vi "Global_params_reg.vi"() -> ()   [LabVIEW 2019]
uses:
  _ctrl/config_aging.ctl
  Setting_reg.ctl
  Breakdown-Spec.ctl
  _ctrl/DL950_config.ctl
  _ctrl/BP4610_config.ctl
  _ctrl/DSP_config.ctl
  Devices/NI Board/cDAQ-9221 AI/Set_NIAI.ctl
  _ctrl/cDAQ-9269 Config.ctl
  Devices/NI Board/cDAQ-9269 AO/Set_AO_Wave-config.ctl
panel:
  in  "Params_reg-all":T10={"Params"={"Setting"={"제어 전압[V]"=0.0, "출력전압[V]"=0.0, "전류[A]"=0.0, "출력전류[A]"=0.0, "ON[초]"=0.0, "OFF[초]"=0.0, "Irms 허용치 from "=0.0, "Irms 허용치 to"=0.0, "AO Delay ms"=0, "Log"=path "", "result"=path ""}, "TestName"="", "Result path"=path "", "파일 생성 주기[N]"=0, "Test Specs"={"제어단 단선 Irms[mA](이하)"=0.0, "제어단 특성 전류 Irms[mA] Max"=0.0, "제어단 특성 전류 Irms[mA] Min"=0.0, "출력단 단선 Irms[mA](이하)"=0.0, "출력단 특성 전류 Irms[mA]  Max"=0.0, "출력단 특성전류 Irms[mA]  Min"=0.0, "온도[degree]"=0.0}}, "DL950_config"={"Timeout"=10000, "Time Div"=19, "Acq Mode"=0, "Record Len"=5, "Record Num"=0, "Start Point"=0, "End Poin"=60000, "Visa"="TCPIP0::192.168.0.100::inst0::INSTR", "Config Voltage"=[{"Enable"=TRUE, "Ch"=0, "V Div"=12, "Coupling"=1, "Probe"=3, "Act.Items"=FALSE, "items"=[]}, {"Enable"=TRUE, "Ch"=0, "V Div"=12, "Coupling"=1, "Probe"=3, "Act.Items"=FALSE, "items"=[]}], "Trigger on"=FALSE, "Trigger Level"=0.0, "Reset"=FALSE, "Config Temp"=[], "Trig Mode"=1, "Trig Pos"=50.0, "Trigger Slope"=0, "Trigger Source "=1, "Trig Start -5"=-5.0, "End 5"=5.0}, "BP4610 Config"={"VISA"="", "Limit-BP"={"Set"=enum."Current", "Voltage+[V]"=20.0, "Current+[A]"=5.0, "Voltage-[V]"=-20.0, "Current-[A]"=-5.0}, "SET BP"={"Set"=enum."FREQ/WAVE", "Operation mode"=0, "Voltage[Vp-p]"=0.0, "Current[Ap-p]"=0.0, "Voltage[V]"=0.0, "Current[A]"=0.0, "Frequency[Hz]"=1.0, "Waveform"=enum."Sine"}}, "DSP1950 Config"={"Port"="TCPIP0::192.168.0.14::HISLIP0::INSTR", "OVP Level"=0.0, "OCP Level"=0.0, "Current"=0.0, "Voltage"=0.0}, "DMM 2470 Config"={"Source Mode"=enum."Voltage", "Source Limit Level"=0.01, "Source Level"=0.0, "Output_2470"=FALSE}, "cDAQ-9221 Config"={"input terminal"=10083, "minimum value"=-60.0, "maximum value"=60.0, "number of samples"=1000, "rate"=10000.0, "sample mode"=10123, "physical channels"=""}, "cDAQ-9467 Config"="", "cDAQ-9269 AO Config"={"Ch"="cDAQ1Mod1/ao0", "Max V"=5.0, "Min V"=-5.0, " Rate"=1000.0, "N pts"=100, "sample mode"=10178}, "AO_Wave-config"={"offset"=0.0, "Samples"=0, "duty"=0.0, "Rate"=0.0, "wfm"={"Freq"=0.0, "Amp"=0.0, "Type"=enum."Sine Wave"}}} {"cDAQ-9269 AO Config"."sample mode" items=["유한 샘플"=10178, "연속 샘플"=10123, "하드웨어 타이밍에 의한 단일 포인트"=12522]; "cDAQ-9221 Config"."sample mode" items=["Finite Samples"=10178, "Continuous Samples"=10123, "Hardware Timed Single Point"=12522]; "cDAQ-9221 Config"."rate" format="%0.2f"; "cDAQ-9221 Config"."maximum value" format="%^.2e"; "cDAQ-9221 Config"."minimum value" format="%^.2e"; "cDAQ-9221 Config"."input terminal" items=["default"=-1, "RSE"=10083, "NRSE"=10078, "Differential"=10106, "Pseudodifferential"=12529]; "DSP1950 Config"."OCP Level" format="%#_13g"; "DSP1950 Config"."OVP Level" format="%#_13g"; "BP4610 Config"."SET BP"."Frequency[Hz]" min=1.0 max=100000.0 step=0.1; "BP4610 Config"."SET BP"."Current[A]" min=-20.0 max=20.0 step=0.001; "BP4610 Config"."SET BP"."Voltage[V]" min=-115.0 max=115.0 step=0.01; "BP4610 Config"."SET BP"."Current[Ap-p]" min=0.0 max=60.0 step=0.01; "BP4610 Config"."SET BP"."Voltage[Vp-p]" min=0.0 max=120.0 step=0.1; "BP4610 Config"."SET BP"."Operation mode" items=["CV-INT", "CV-EXT", "CV-ADD", "CC-INT", "CC-EXT", "CC-ADD"]; "BP4610 Config"."Limit-BP"."Current-[A]" min=-20.0 max=20.0 step=0.001; "BP4610 Config"."Limit-BP"."Voltage-[V]" min=-115.0 max=115.0 step=0.01; "BP4610 Config"."Limit-BP"."Current+[A]" min=0.0 max=60.0 step=0.01; "BP4610 Config"."Limit-BP"."Voltage+[V]" min=0.0 max=120.0 step=0.1; "DL950_config"."End 5" format="%.2g"; "DL950_config"."Trig Start -5" format="%.2f"; "DL950_config"."Trigger Source" items=["", "CH1", "CH2", "CH3", "CH4", "CH5", "CH6", "CH7", "CH8", "CH9", "CH10", "CH11", "CH12", "CH13", "CH14", "CH15", "CH16", "RMATH1", "RMATH2", "RMATH3", "RMATH4", "RMATH5", "RMATH6", "RMATH7", "RMATH8", "RMATH9", "RMATH10", "RMATH11", "RMATH12", "RMATH13", "RMATH14", "RMATH15", "RMATH16"]; "DL950_config"."Trigger Slope" items=["Rising", "Falling", "Both"]; "DL950_config"."Trig Pos" format="%.1f"; "DL950_config"."Trig Mode" items=["Normal", "Auto", "Auto Level", "Single", "Single(N)", "On Start", "No Set"]; "DL950_config"."Config Temp"."Type" items=["K", "E", "J", "T", "L", "U", "N", "R", "S", "B", "W", "Au7fe"]; "DL950_config"."Config Temp"."Channel" items=["", "CH1", "CH2", "CH3", "CH4", "CH5", "CH6", "CH7", "CH8", "CH9", "CH10", "CH11", "CH12", "CH13", "CH14", "CH15", "CH16"]; "DL950_config"."Trigger Level" format="%.3p"; "DL950_config"."Config Voltage"."items" items=["Peak to Peak", "Amplitude", "Max", "Min", "High", "Low", "Average", "Middle", "Rms", "Standard Deviation", "+Overshoot", "-Overshoot", "Rise", "Fall", "Frequency", "Period", "+Width", "-Width", "Duty Cycle", "Pulse Count", "Burst1 Width", "Burst2 Width", "Average Frequency", "Average Period", "Int1TY", "Int2TY"]; "DL950_config"."Config Voltage"."Probe" items=["1:1", "2:1", "5:1", "10:1", "20:1", "50:1", "100:1", "200:1", "500:1", "1000:1", "2000:1", "5000:1", "10k:1", "20k:1", "50k:1", "0.1A:1V", "0.2A:1V", "0.5A:1V", "1A:1V", "2A:1V", "5A:1V", "10A:1V", "20A:1V", "50A:1V", "100A:1V", "200A:1V", "250A:1V", "400A:1V", "500A:1V", "1kA:1V", "2kA:1V", "5kA:1V", "10kA:1V", "20kA:1V", "50kA:1V", "NoSet"]; "DL950_config"."Config Voltage"."Ch" items=["None", "CH1", "CH2", "CH3", "CH4", "CH5", "CH6", "CH7", "CH8", "CH9", "CH10", "CH11", "CH12", "CH13", "CH14", "CH15", "CH16", "MATH1", "MATH2", "MATH3", "MATH4", "MATH5", "MATH6", "MATH7", "MATH8", "EVENT"]; "DL950_config"."Config Voltage"."Coupling" items=["AC", "DC", "Ground", "AC-RMS", "DC-RMS"]; "DL950_config"."Config Voltage"."V Div" items=["0.1m", "0.2m", "0.5m", "1m", "2m", "5m", "10m", "20m", "50m", "100m", "200m", "500m", "1", "2", "4", "5", "8", "10", "20", "40", "50", "80", "100", "200", "400", "500", "800", "1k", "2k", "4k", "5k", "8k", "10k", "20k", "25k", "50k", "100k", "250k", "500k", "1000k"]; "DL950_config"."Record Len" items=["10k", "25k", "50k", "100k", "250k", "500k", "1M", "2.5M", "5M", "10M", "25M", "50M", "100M", "250M", "500M", "1G", "2G", "4G", "5G", "10G", "20G", "50G"]; "DL950_config"."Acq Mode" items=["Normal", "Average", "Envelope"]; "DL950_config"."Time Div" items=["100ns", "200ns", "500ns", "1us", "2us", "5us", "10us", "20us", "50us", "100us", "200us", "500us", "1ms", "2ms", "5ms", "10ms", "20ms", "50ms", "100ms", "200ms", "500ms", "1s", "2s", "3s", "4s", "5s", "6s", "10s", "20s", "30s", "1min", "2min", "3min", "4min", "5min", "6min", "10min", "12min", "30min", "1hour", "2hour", "3hour", "4hour", "5hour", "6hour", "8hour", "10hour", "12hour", "1day", "2day", "3day", "4day", "5day"]; "Params"."Test Specs"."출력단 특성전류 Irms[mA]  Min" format="%#.2f"; "Params"."Test Specs"."출력단 특성 전류 Irms[mA]  Max" format="%#.2f"; "Params"."Test Specs"."출력단 단선 Irms[mA](이하)" format="%#.2f"; "Params"."Test Specs"."제어단 특성 전류 Irms[mA] Min" format="%#.2f"; "Params"."Test Specs"."제어단 특성 전류 Irms[mA] Max" format="%#.2f"; "Params"."Test Specs"."제어단 단선 Irms[mA](이하)" format="%#.2f"}
  # "제어단"
  # "출력단"
  # "온도기준"
  # "Highpower"
  # "Control"
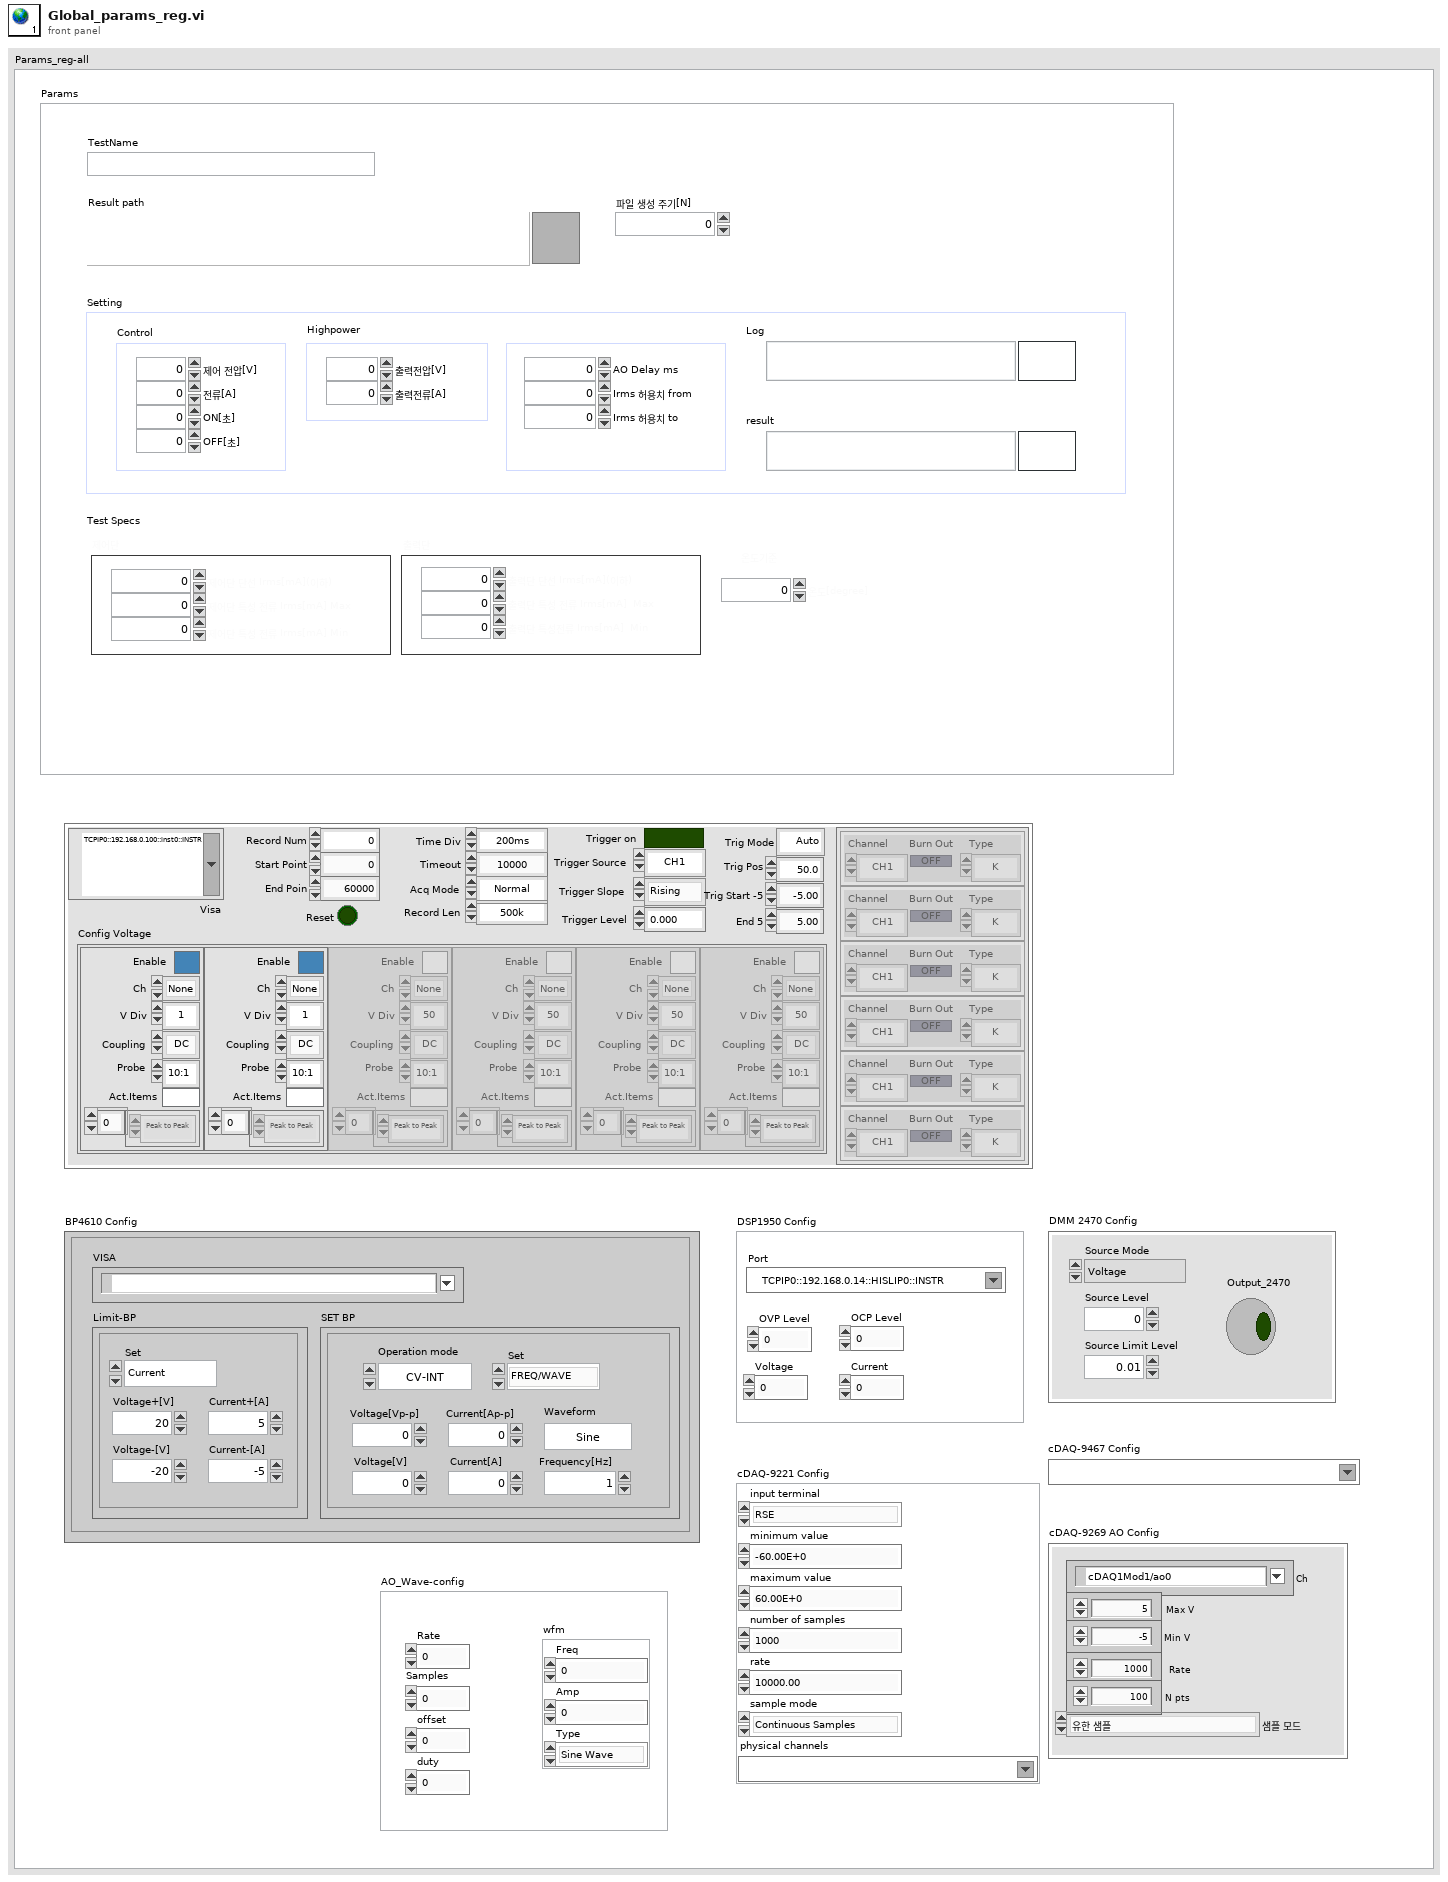
[diagram p1: front panel]
types:
  T1 = typedef "config_aging.ctl" = cluster{"Setting":T2, "TestName":string, "Result path":path, "파일 생성 주기[N]":u8, "Test Specs":T3}
  T2 = typedef "Setting_reg.ctl" = cluster{"제어 전압[V]":dbl, "출력전압[V]":dbl, "전류[A]":dbl, "출력전류[A]":dbl, "ON[초]":dbl, "OFF[초]":dbl, "Irms 허용치 from ":dbl, "Irms 허용치 to":dbl, "AO Delay ms":u32, "Log":path, "result":path}
  T3 = typedef "Breakdown-Spec.ctl" = cluster{"제어단 단선 Irms[mA](이하)":dbl, "제어단 특성 전류 Irms[mA] Max":dbl, "제어단 특성 전류 Irms[mA] Min":dbl, "출력단 단선 Irms[mA](이하)":dbl, "출력단 특성 전류 Irms[mA]  Max":dbl, "출력단 특성전류 Irms[mA]  Min":dbl, "온도[degree]":dbl}
  T4 = typedef "DL950_config.ctl" = cluster{"Timeout":u32, "Time Div":i32, "Acq Mode":i32, "Record Len":i32, "Record Num":i32, "Start Point":i64, "End Poin":i64, "Visa":refnum<visa-resource-name>, "Config Voltage":cluster{"Enable":bool, "Ch":u16, "V Div":i32, "Coupling":i32, "Probe":i32, "Act.Items":bool, "items":i32[]}[], "Trigger on":bool, "Trigger Level":dbl, "Reset":bool, "Config Temp":cluster{"Channel":u16, "Burn Out":bool, " Type ":i32}[], "Trig Mode":i32, "Trig Pos":dbl, "Trigger Slope":i32, "Trigger Source ":i32, "Trig Start -5":dbl, "End 5":dbl}
  T5 = typedef "BP4610_config.ctl" = cluster{"VISA":refnum<visa-resource-name>, "Limit-BP":cluster{"Set":enum16{"Current", "Voltage"}, "Voltage+[V]":dbl, "Current+[A]":dbl, "Voltage-[V]":dbl, "Current-[A]":dbl}, "SET BP":cluster{"Set":enum16{"Current", "Voltage", "FREQ/WAVE"}, "Operation mode":u16, "Voltage[Vp-p]":dbl, "Current[Ap-p]":dbl, "Voltage[V]":dbl, "Current[A]":dbl, "Frequency[Hz]":dbl, "Waveform":enum16{"Sine", "Square", "ARB 1", "ARB 2", "ARB 3", "ARB 4", "ARB 5", "ARB 6", "ARB 7", "ARB 8", "ARB 9", "ARB 10", "ARB 11", "ARB 12", "ARB 13", "ARB 14", "ARB 15", "ARB 16"}}}
  T6 = typedef "DSP_config.ctl" = cluster{"Port":refnum<visa-resource-name>, "OVP Level":dbl, "OCP Level":dbl, "Current":dbl, "Voltage":dbl}
  T7 = typedef "Set_NIAI.ctl" = cluster{"input terminal":i32, "minimum value":dbl, "maximum value":dbl, "number of samples":i32, "rate":dbl, "sample mode":i32, "physical channels":tag}
  T8 = typedef "cDAQ-9269 Config.ctl" = cluster{"Ch":tag, "Max V":dbl, "Min V":dbl, " Rate":dbl, "N pts":i32, "sample mode":i32}
  T9 = typedef "Set_AO_Wave-config.ctl" = cluster{"offset":dbl, "Samples":i32, "duty":dbl, "Rate":dbl, "wfm":cluster{"Freq":dbl, "Amp":dbl, "Type":enum16{"Sine Wave", "Triangle Wave", "Square Wave", "Sawtooth Wave"}}}
  T10 = cluster{"Params":T1, "DL950_config":T4, "BP4610 Config":T5, "DSP1950 Config":T6, "DMM 2470 Config":cluster{"Source Mode":enum16{"Voltage", "Current"}, "Source Limit Level":dbl, "Source Level":dbl, "Output_2470":bool}, "cDAQ-9221 Config":T7, "cDAQ-9467 Config":tag, "cDAQ-9269 AO Config":T8, "AO_Wave-config":T9}
diagram:
